vi "Write Target.vi"(8 "error in (no error)":errorcluster, 10 "Target":u32, 11 "Simple Linked List Task in":refnum<class "Simple Linked List Task.lvclass">) -> (0 "error out":errorcluster, 3 "Simple Linked List Task out":refnum<class "Simple Linked List Task.lvclass">)   [LabVIEW 2024, in "Simple Linked List Task.lvclass"]
uses:
  Simple Linked List Task.lvclass
  Simple Linked List Task.lvclass/Simple Linked List Task.ctl
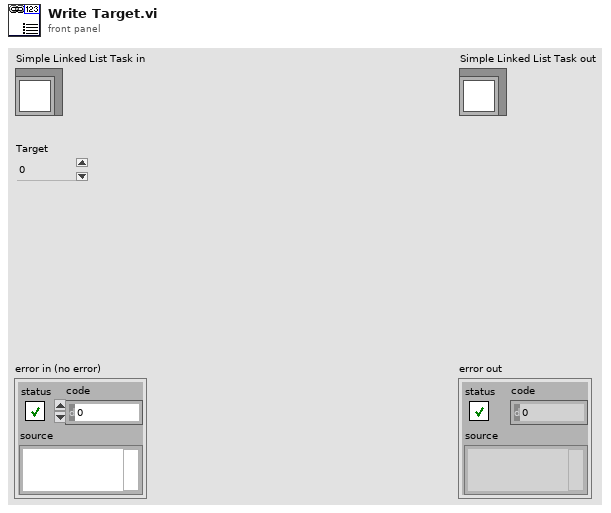
[diagram p1: front panel]
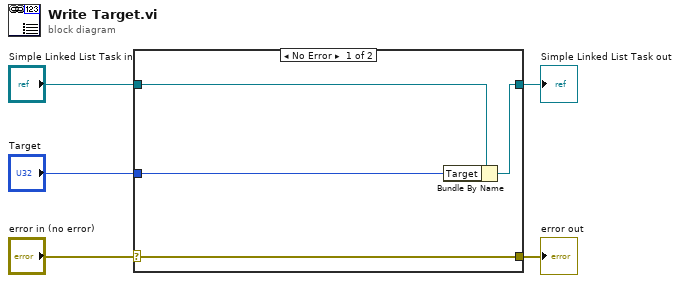
[diagram p0: block diagram]
diagram:
  n1 = case shown="No Error" "error in (no error)" {
    selector: "error in (no error)" -> [w9 w10]
    tunnel: [w9 w10] -> w4
    tunnel: [w7 w11] -> w2
    tunnel: "Simple Linked List Task in" -> [w8 w11]
    tunnel: "Target" -> [w6 _]
    frame No Error {
      n2 = Bundle By Name(cluster=w8, "Target"=w6) -> (w7:refnum<class "Simple Linked List Task.lvclass">)
    }
    frame Error {
    }
  }
  "error out" <- w4
  "Simple Linked List Task out" <- w2
